vi "Read UID.vi"(11 "Event Transport in":refnum<class "Event Transport.lvclass">) -> (2 "UID":i32)   [LabVIEW 2020, in "jettl.lvlib" / "Event Transport.lvlib" / "Event Transport.lvclass"]
uses:
  Event Transport.lvclass
  Event Transport.lvclass/Event Transport.ctl
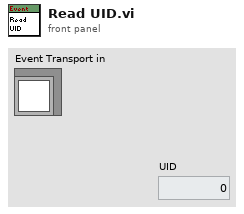
[diagram p1: front panel]
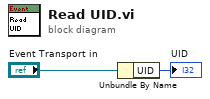
[diagram p0: block diagram]
diagram:
  n1 = Unbundle By Name("Event Transport in") -> ("UID"=→"UID":i32)
